vi "Get Column Name Query SQLServer.vi"(8 "error in (no error)":errorcluster, 10 "Table Name":string, 11 "ADODB._Connection":refnum<k7>) -> (0 "error out":errorcluster, 2 "Selected Data":string[][](array[string]), 3 "ADODB._Connection 2":refnum<k7>)   [LabVIEW 2017]
panel:
  out "Query":string
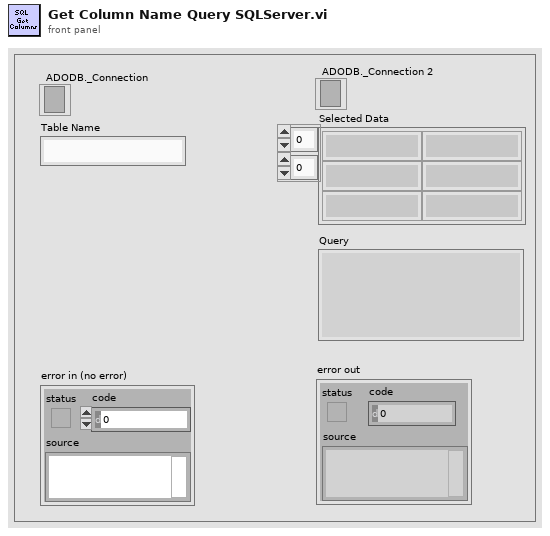
[diagram p1: front panel]
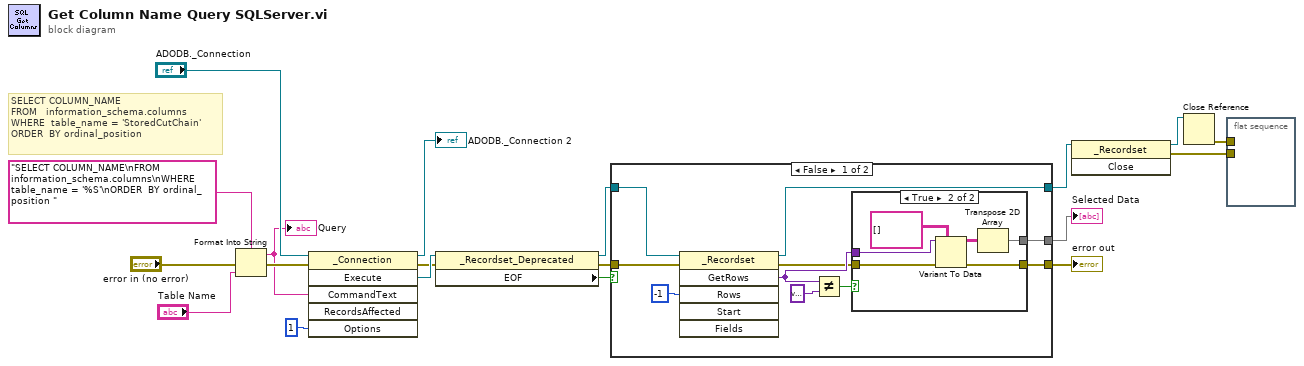
[diagram p0: block diagram]
diagram:
  # "SELECT COLUMN_NAME\nFROM   information_schema.columns\nWHERE  table_name = 'StoredCutChain'\nORDER  BY ordinal_position"
  n1 = Format Into String(format string="SELECT COLUMN_NAME\nFROM   information_schema.columns\nWHERE  table_name = '%S'\nORDER  BY ordinal_position " ("CommandText"), error in="error in (no error)", "Table Name") -> (resulting string=w3:string, error out=w15:errorcluster)  [unwired: 1 in]
  "Query" <- w3
  n2 = invoke class="_Connection" method="Execute"(reference="ADODB._Connection", error in=w15, "CommandText"=w3, "Options"=1) -> (reference out=→"ADODB._Connection 2":refnum<k7>, error out=w12:errorcluster, "Execute"=w13:refnum<k7>)  [unwired: 2 in, 3 out]
  n3 = property class="_Recordset_Deprecated"(reference=w13, error in=w12) -> (reference out=w9:refnum<k7>, error out=w11:errorcluster, "EOF"=w10:bool)
  n4 = case shown="False" w10 {
    tunnel: [w29 _] -> w6
    tunnel: [w28 _] -> w1
    tunnel: w9 -> [w23 w37]
    tunnel: w11 -> [w22 _]
    tunnel: [w20 w37] -> w8
    frame False {
      n5 = invoke class="_Recordset" method="GetRows"(reference=w23, error in=w22, "Rows"=-1) -> (reference out=w20:refnum<k7>, error out=w21:errorcluster, "GetRows"=w24:variant)  [unwired: 3 in, 3 out]
      n6 = Not Equal?(x=w24, y=variant) -> (x != y?=w25:bool)
      n7 = case shown="True" w25 {
        tunnel: w24 -> [_ w35]
        tunnel: w21 -> [w30 w36]
        tunnel: [w30 w33] -> w29
        tunnel: [_ w31] -> w28
        frame False {
        }
        frame True {
          n8 = Variant To Data(error in=w36, type=string[][] [], Variant=w35) -> (data=w32:string[][], error out=w33:errorcluster)
          n9 = Transpose 2D Array(2D array=w32) -> (transposed array=w31:string[][])
        }
      }
    }
    frame True {
    }
  }
  "error out" <- w6
  "Selected Data" <- w1
  n10 = invoke class="_Recordset" method="Close"(reference=w8) -> (reference out=w5:refnum<k7>, error out=w7:errorcluster)  [unwired: 2 in, 1 out]
  n11 = Close Reference(reference=w5) -> (error out=w4:errorcluster)  [unwired: 1 in]
  n12 = flat-sequence {
    tunnel: w7 -> [_]
    tunnel: w4 -> [_]
    frame #0 {
    }
  }
